vi "Write Config Refnum.vi"(10 "config data":T1, 11 "Configurations in":refnum<class "Configurations.lvclass">) -> (3 "Configurations out":refnum<class "Configurations.lvclass">)   [LabVIEW 2016, in "Configurations.lvlib" / "Configurations.lvclass"]
uses:
  Configurations.lvclass
  <vilib>/Utility/config.llb/Config Data RefNum.ctl
  Configurations.lvclass/Configurations.ctl
  <vilib>/Utility/config.llb/NI_LVConfig.lvlib
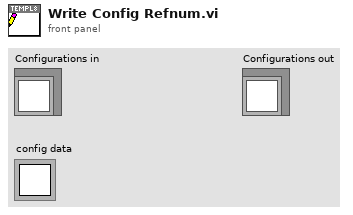
[diagram p1: front panel]
types:
  T1 = typedef "NI_LVConfig.lvlib/Config Data RefNum.ctl" = refnum<k1>
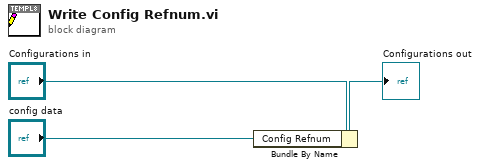
[diagram p0: block diagram]
diagram:
  n1 = Bundle By Name(cluster="Configurations in", "Config Refnum"="config data") -> (→"Configurations out":refnum<class "Configurations.lvclass">)
